vi "Obs_move.vi"(4 "Reset_x":i32, 6 "Return_x":i32, 7 "Mov_Spd":i32, 8 "error in":errorcluster, 10 "Obst D_REF":refnum<vi>[](array[refnum]), 11 "Obst U_Ref":refnum<vi>[](array[refnum])) -> (0 "error out":errorcluster)   [LabVIEW 8.6]
panel:
  # "障礙物重置的位置必須考慮其\n寬度、間距和移動速度\n不然可能會重疊或看起來不協調"
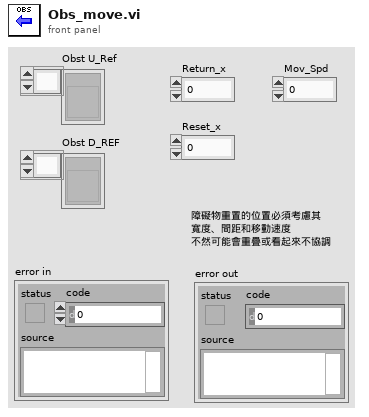
[diagram p1: front panel]
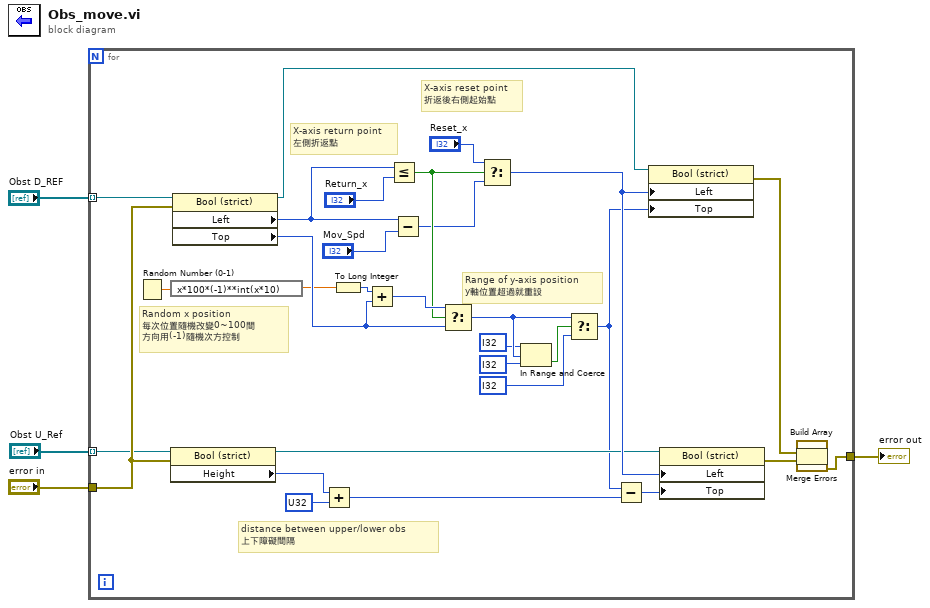
[diagram p0: block diagram]
diagram:
  n1 = for {
    tunnel: [w18] -> w4
    tunnel: "error in" -> [w15]
    tunnel: "Obst U_Ref" -> [w14] mode=indexing
    tunnel: "Obst D_REF" -> [w13] mode=indexing
    # "Range of y-axis position\ny軸位置超過就重設"
    # "Random x position\n每次位置隨機改變0~100間\n方向用(-1)隨機次方控制"
    # "X-axis return point\n左側折返點"
    # "X-axis reset point\n折返後右側起始點"
    # "distance between upper/lower obs\n上下障礙間隔"
    n2 = Random Number (0-1)() -> (number: 0 to 1=w24:dbl)
    n3 = expression code="x*100*(-1)**int(x*10)"(w24) -> (w26:dbl)
    n4 = property on="Property Node" class="Bool (strict)"(reference=w14, error in=w15) -> (reference out=w20:refnum<vi>, "Height"=w32:u32)  [unwired: 1 out]
    n5 = property on="Property Node" class="Bool (strict)"(reference=w13, error in=w15) -> (reference out=w19:refnum<vi>, "Left"=w30:i32, "Top"=w28:i32)  [unwired: 1 out]
    n6 = Add(x=w32, y=u32 ?) -> (x+y=w12:u32)
    n7 = To Long Integer(number=w26) -> (32bit integer=w25:i32)
    n8 = Add(x=w25, y=w28) -> (x+y=w27:i32)
    n9 = Less Or Equal?(x=w30, y="Return_x") -> (x <= y?=w23:bool)
    n10 = Subtract(x=w30, y="Mov_Spd") -> (x-y=w21:i32)
    n11 = Select(t=w27, s=w23, f=w28) -> (s? t:f=w8:i32)
    n12 = Select(t="Reset_x", s=w23, f=w21) -> (s? t:f=w35:i32)
    n13 = In Range and Coerce(upper limit=i32 ? ("y"), x=w8, lower limit=i32 ? ("y")) -> (In Range?=w11:bool)  [unwired: 1 out]
    n14 = Select(t=w8, s=w11, f=i32 ? ("y")) -> (s? t:f=w9:i32)
    n15 = Subtract(x=w9, y=w12) -> (x-y=w34:u32)
    n16 = property on="Property Node" class="Bool (strict)"(reference=w19, "Left"=w35, "Top"=w9) -> (error out=w16:errorcluster)  [unwired: 1 in, 1 out]
    n17 = property on="Property Node" class="Bool (strict)"(reference=w20, "Left"=w35, "Top"=w34) -> (error out=w17:errorcluster)  [unwired: 1 in, 1 out]
    n18 = Build Array(w16, w17) -> (w5:errorcluster[])
    n19 = call <vilib>:"Merge Errors.vi"("error array in"=w5) -> ("error out"=w18:errorcluster)  [unwired: 6 in]
  }
  "error out" <- w4
